vi "Test Monitor.vi"() -> ()   [LabVIEW 2015]
panel:
  in  "Points":i32=10
  in  "Process Stop Button":bool
  in  "Replot":bool
  out "XY Graph":cluster{dbl[], dbl[]}(graph)
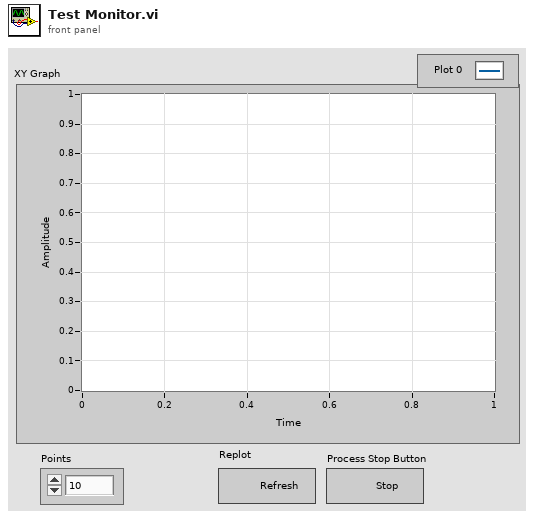
[diagram p1: front panel]
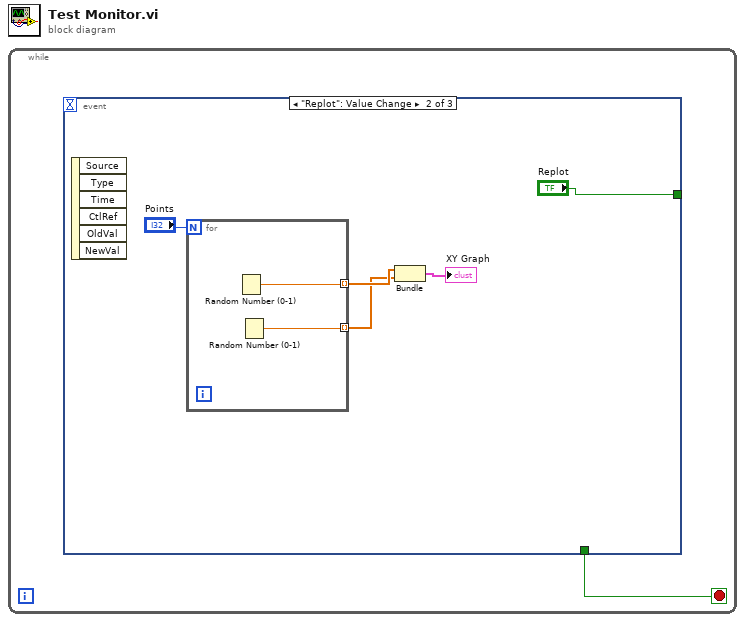
[diagram p0: block diagram]
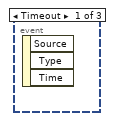
[diagram p2: hidden frame]
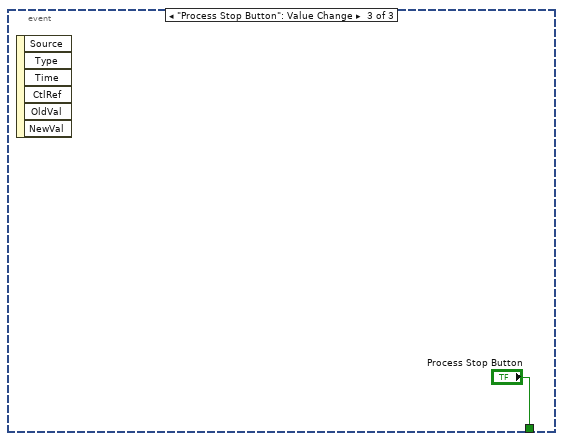
[diagram p3: hidden frame]
diagram:
  n1 = while {
    stop <- w1 stop-if-true
    n2 = event shown="[1] \"Replot\": Value Change" {
      selector: _ -> [_ _ _]
      dyn-events: _ -> [_ _ _]
      timeout: _ -> [_ _ _]
      tunnel: [_ "Replot" _] -> _
      tunnel: [_ _ "Process Stop Button"] -> w1
      event Timeout {
        n3 = event-data() -> ()  [unwired: 1 in, 3 out]
      }
      event "Replot": Value Change {
        n4 = event-data() -> ()  [unwired: 1 in, 6 out]
        n5 = for {
          N: "Points" -> [_]
          tunnel: [w8] -> w4 mode=indexing
          tunnel: [w7] -> w3 mode=indexing
          n6 = Random Number (0-1)() -> (number: 0 to 1=w8:dbl)
          n7 = Random Number (0-1)() -> (number: 0 to 1=w7:dbl)
        }
        n8 = Bundle(w4, w3) -> (→"XY Graph":cluster{dbl[], dbl[]})  [unwired: 1 in]
      }
      event "Process Stop Button": Value Change {
        n9 = event-data() -> ()  [unwired: 1 in, 6 out]
      }
    }
  }
